vi "MGI Match Element in String.vi"(5 "Precedence (Index)":T1, 7 "Match Pattern? (F)":bool, 9 "Match[]":string[](array[string]), 10 "Offset in":i32, 11 "String":string) -> (1 "Index":i32, 2 "Offset past match":i32, 3 "Match":string)   [LabVIEW 2020]
doc: "This VI searches <B>String</B> at <B>Offset in<B> for an occurence of one of the elements of <B>Match[]</B>. If no match is found, then <B>Offset past match</B> and <B>Index</B> are -1, and <B>Match</B> is empty.\n<B>Precedence</B> determines result if multple matches exist. For example:\nString=A B C\nMatch[] = {C, A}\nIf <B>Precedence</B> is Offset, then \"A\" is output. If it is Index, then \"C\" is output.\n\nAuthored by Shawn Walpole\nsupport@mooregoodideas.com\nwww.mooregoodideas.com\n\nCopyright (c) 2010, Moore Good Ideas, Inc.\n\nAll rights reserved.\n\nRedistribution and use in source and binary forms, with or without modification, are permitted provided that the following conditions are met:\n\n * Redistributions of source code must retain the above copyright notice, this list of conditions and the following disclaimer.\n * Redistributions in binary form must reproduce the above copyright notice, this list of conditions and the following disclaimer in the documentation and/or other materials provided with the distribution.\n * Neither the name of Moore Good Ideas, Inc. nor the names of its contributors may be used to endorse or promote products derived from this software without specific prior written permission.\n\nTHIS SOFTWARE IS PROVIDED BY THE COPYRIGHT HOLDERS AND CONTRIBUTORS \"AS IS\" AND ANY EXPRESS OR IMPLIED WARRANTIES, INCLUDING, BUT NOT LIMITED TO, THE IMPLIED WARRANTIES OF MERCHANTABILITY AND FITNESS FOR A PARTICULAR PURPOSE ARE DISCLAIMED. IN NO EVENT SHALL THE COPYRIGHT OWNER OR CONTRIBUTORS BE LIABLE FOR ANY DIRECT, INDIRECT, INCIDENTAL, SPECIAL, EXEMPLARY, OR CONSEQUENTIAL DAMAGES (INCLUDING, BUT NOT LIMITED TO, PROCUREMENT OF SUBSTITUTE GOODS OR SERVICES; LOSS OF USE, DATA, OR PROFITS; OR BUSINESS INTERRUPTION) HOWEVER CAUSED AND ON ANY THEORY OF LIABILITY, WHETHER IN CONTRACT, STRICT LIABILITY, OR TORT (INCLUDING NEGLIGENCE OR OTHERWISE) ARISING IN ANY WAY OUT OF THE USE OF THIS SOFTWARE, EVEN IF ADVISED OF THE POSSIBILITY OF SUCH DAMAGE."
uses:
  <userlib>/_MGI/String/MGI Match Precedence Enum.ctl
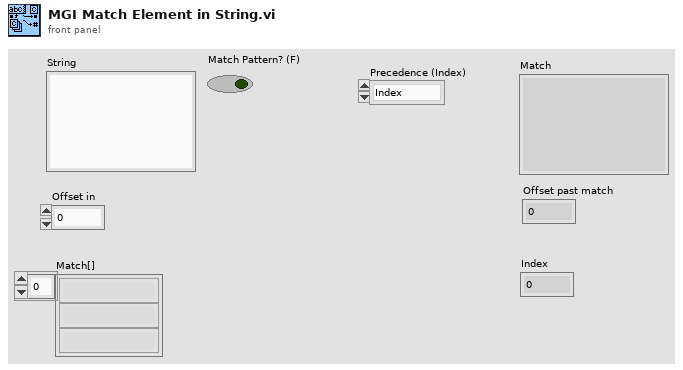
[diagram p1: front panel]
types:
  T1 = typedef "MGI Match Precedence Enum.ctl" = enum16{"Index", "Offset"}
  T2 = cluster{"offset past match":i32, "offset past match":i32, i32, "String":string}
  T3 = cluster{"offset past match":i32, "offset past match":i32, i32, "String":string}[]
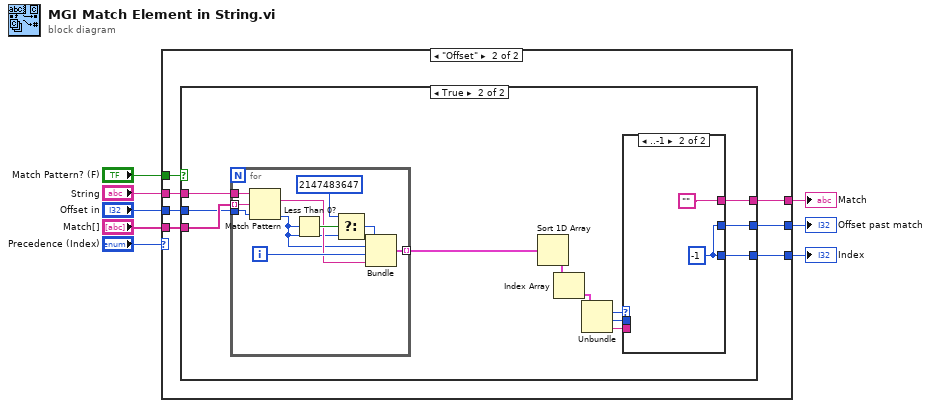
[diagram p0: block diagram]
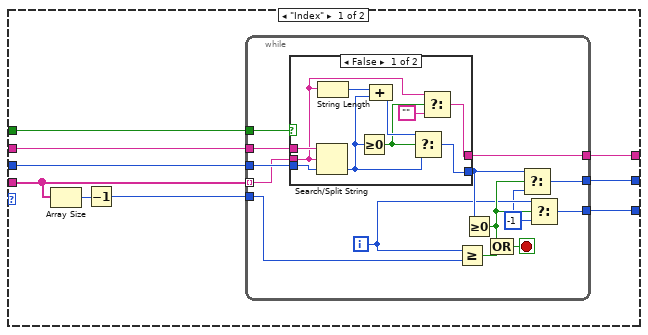
[diagram p2: hidden frame]
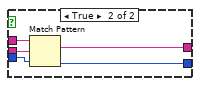
[diagram p3: hidden frame]
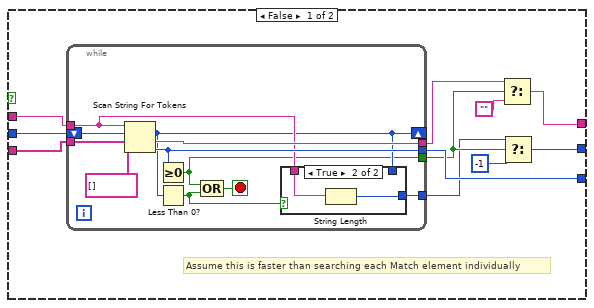
[diagram p4: hidden frame]
diagram:
  n1 = case shown="\"Offset\"" "Precedence (Index)" {
    tunnel: "String" -> [w15 w53]
    tunnel: [w10 w52] -> w3
    tunnel: "Match[]" -> [w17 w51]
    tunnel: [w12 w50] -> w5
    tunnel: "Offset in" -> [w16 w49]
    tunnel: [w11 w48] -> w4
    tunnel: "Match Pattern? (F)" -> [w9 w47]
    frame "Index" {
      n2 = Array Size(array=w17) -> (size(s)=w14:i32)
      n3 = Decrement(x=w14) -> (x-1=w13:i32)
      n4 = while {
        tunnel: w15 -> [w31]
        tunnel: w16 -> [w23]
        tunnel: w17 -> [w19] mode=indexing
        tunnel: w13 -> [w30]
        tunnel: [w27] -> w12
        tunnel: [w24] -> w11
        tunnel: [w21] -> w10
        tunnel: w9 -> [w20]
        i -> [w22]
        stop <- w28 stop-if-true
        w18 = -1 ("f")
        n5 = case shown="False" w20 {
          tunnel: w31 -> [w41 w46]
          tunnel: w19 -> [w33 w45]
          tunnel: [w32 w44] -> w27
          tunnel: [w36 w43] -> w25
          tunnel: w23 -> [w40 w42]
          frame False {
            n6 = Search/Split String(string=w41, search string/char (-)=w33, offset (0)=w40) -> (offset of match=w37:i32)  [unwired: 2 out]
            n7 = String Length(string=w33) -> (length=w39:i32)
            n8 = Greater Or Equal To 0?(x=w37) -> (x >= 0?=w35:bool)
            n9 = Compound Arithmetic op=ADD(w39, w37) -> (w38:i32)
            n10 = Select(t=w38, s=w35, f=w37) -> (s? t:f=w36:i32)
            n11 = Select(t=w33, s=w35, f="") -> (s? t:f=w32:string)
          }
          frame True {
            n12 = Match Pattern(string=w46, regular expression=w45, offset (0)=w42) -> (match substring=w44:string, offset past match=w43:i32)  [unwired: 2 out]
          }
        }
        n13 = Greater Or Equal?(x=w22, y=w30) -> (x >= y?=w29:bool)
        n14 = Greater Or Equal To 0?(x=w25) -> (x >= 0?=w26:bool)
        n15 = Compound Arithmetic op=OR(w26, w29) -> (w28:bool)
        n16 = Select(t=w25, s=w26, f=w18) -> (s? t:f=w24:i32)
        n17 = Select(t=w22, s=w26, f=w18) -> (s? t:f=w21:i32)
      }
    }
    frame "Offset" {
      n18 = case shown="True" w47 {
        tunnel: w53 -> [w64 w88]
        tunnel: [w63 w85] -> w52
        tunnel: w51 -> [w62 w90]
        tunnel: [w60 w87] -> w50
        tunnel: w49 -> [w58 w89]
        tunnel: [w57 w86] -> w48
        frame False {
          # "Assume this is faster than searching each Match element individually"
          n19 = while {
            tunnel: w64 -> [w69]
            tunnel: [w73] -> w59
            tunnel: [w71] -> w63
            tunnel: w62 -> [w75]
            shift-right: [w67] -> _
            shift-left: w58 -> [w72]
            tunnel: [w65] -> w61
            tunnel: [w68] -> w54
            stop <- w66 stop-if-true
            n20 = Scan String For Tokens(6:string[] [] ("delimiters (\\s,\\t,\\r,\\n)"), 7:w75, 8:w72, 9:w69) -> (0:w71:i32, 1:w73:string, 2:w67:i32)  [unwired: 2 in, 1 out]
            n21 = Greater Or Equal To 0?(x=w71) -> (x >= 0?=w65:bool)
            n22 = Less Than 0?(x=w67) -> (x < 0?=w70:bool)
            n23 = Compound Arithmetic op=OR(w65, w70) -> (w66:bool)
            n24 = case shown="True" w70 {
              tunnel: w69 -> [_ w78]
              tunnel: [w76 w77] -> w68
              tunnel: w67 -> [w76 _]
              frame False {
              }
              frame True {
                n25 = String Length(string=w78) -> (length=w77:i32)
              }
            }
          }
          n26 = Select(t=w59, s=w61, f="") -> (s? t:f=w60:string)
          n27 = Select(t=w54, s=w61, f=-1) -> (s? t:f=w57:i32)
        }
        frame True {
          n28 = for {
            tunnel: w88 -> [w105]
            tunnel: w89 -> [w102]
            tunnel: w90 -> [w104] mode=indexing
            tunnel: [w97] -> w84 mode=indexing
            i -> [w99]
            n29 = Match Pattern(string=w105, regular expression=w104, offset (0)=w102) -> (match substring=w98:string, offset past match=w96:i32)  [unwired: 2 out]
            n30 = Less Than 0?(x=w96) -> (x < 0?=w103:bool)
            n31 = Select(t=2147483647 ("f"), s=w103, f=w96) -> (s? t:f=w100:i32)
            n32 = Bundle("offset past match"=w100, "offset past match"=w96, w99, "String"=w98) -> (w97:T2)  [unwired: 1 in]
          }
          n33 = Sort 1D Array(array=w84) -> (sorted array=w83:T3)
          n34 = Index Array(array=w83) -> (element=w82:T2)  [unwired: 1 in]
          n35 = Unbundle(w82) -> ("offset past match"=w81:i32, w79:i32, "String"=w80:string)  [unwired: 1 out]
          n36 = case shown="..-1" w81 {
            selector: w81 -> [w93 _]
            tunnel: [w93 w94] -> w86
            tunnel: [w92 ""] -> w87
            tunnel: [w91 w94] -> w85
            tunnel: w80 -> [w92 _]
            tunnel: w79 -> [w91 _]
            frame 0.. {
            }
            frame ..-1 {
              w94 = -1 ("f")
            }
          }
        }
      }
    }
  }
  "Offset past match" <- w4
  "Index" <- w3
  "Match" <- w5
